vi "Cal.vi"() -> ()   [LabVIEW 2016]
panel:
  in  "退出":bool
  out "String":string
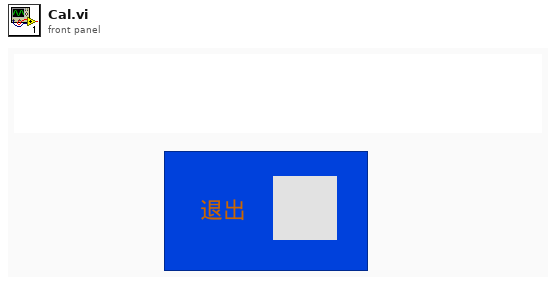
[diagram p1: front panel]
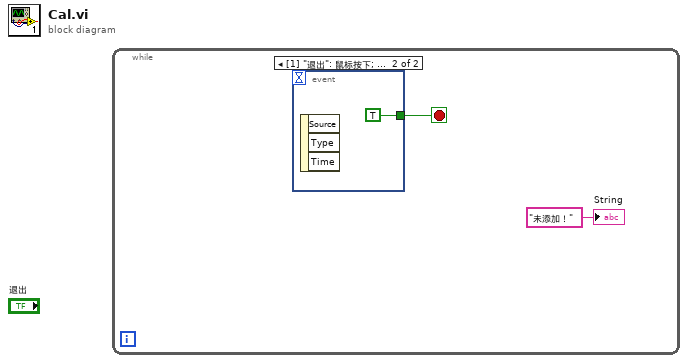
[diagram p0: block diagram]
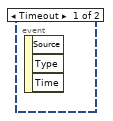
[diagram p2: hidden frame]
diagram:
  n1 = while {
    stop <- w2 stop-if-true
    n2 = event shown="[1] \"退出\": 鼠标按下;  前面板关闭" {
      selector: _ -> [_ _]
      dyn-events: _ -> [_ _]
      timeout: _ -> [_ _]
      tunnel: [_ TRUE] -> w2
      event Timeout {
        n3 = event-data() -> ()  [unwired: 1 in, 3 out]
      }
      event "退出": Mouse Down; Panel Close {
        n4 = event-data() -> ()  [unwired: 1 in, 3 out]
      }
    }
    "String" <- "未添加！" ("String")
  }
